vi "Write Signal Generator.lvclass.vi"(10 "Signal Generator.lvclass":refnum<class "Signal Generator.lvclass">, 11 "Switching Time in":refnum<class "Switching Time.lvclass">) -> (3 "Switching Time out":refnum<class "Switching Time.lvclass">)   [LabVIEW 2020, in "Switching Time.lvclass"]
uses:
  Switching Time.lvclass
  Instruments/Signal Generator/Signal Generator.lvclass
  Switching Time.lvclass/Switching Time.ctl
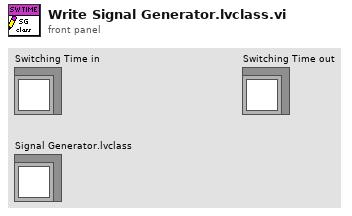
[diagram p1: front panel]
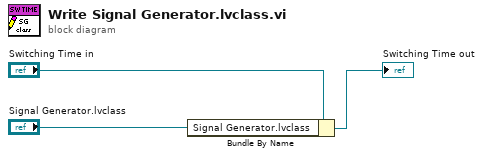
[diagram p0: block diagram]
diagram:
  n1 = Bundle By Name(cluster="Switching Time in", "Signal Generator.lvclass"="Signal Generator.lvclass") -> (→"Switching Time out":refnum<class "Switching Time.lvclass">)
